vi "add wait(SubVI).vi"(10 "字符串":string) -> (1 "ok or cancel":bool, 2 "连接的字符串":string)   [LabVIEW 2019, in "SubVI.lvlib"]
uses:
  SubVI.lvlib
panel:
  in  "cancel":bool
  in  "ok":bool
  in  "Delay(secs)":dbl
  in  "Chamber":bool
  in  "Position":bool
  in  "Field":bool
  in  "Temperature":bool
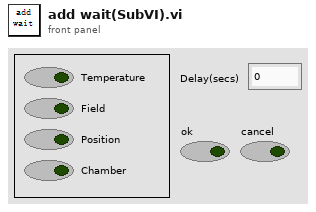
[diagram p1: front panel]
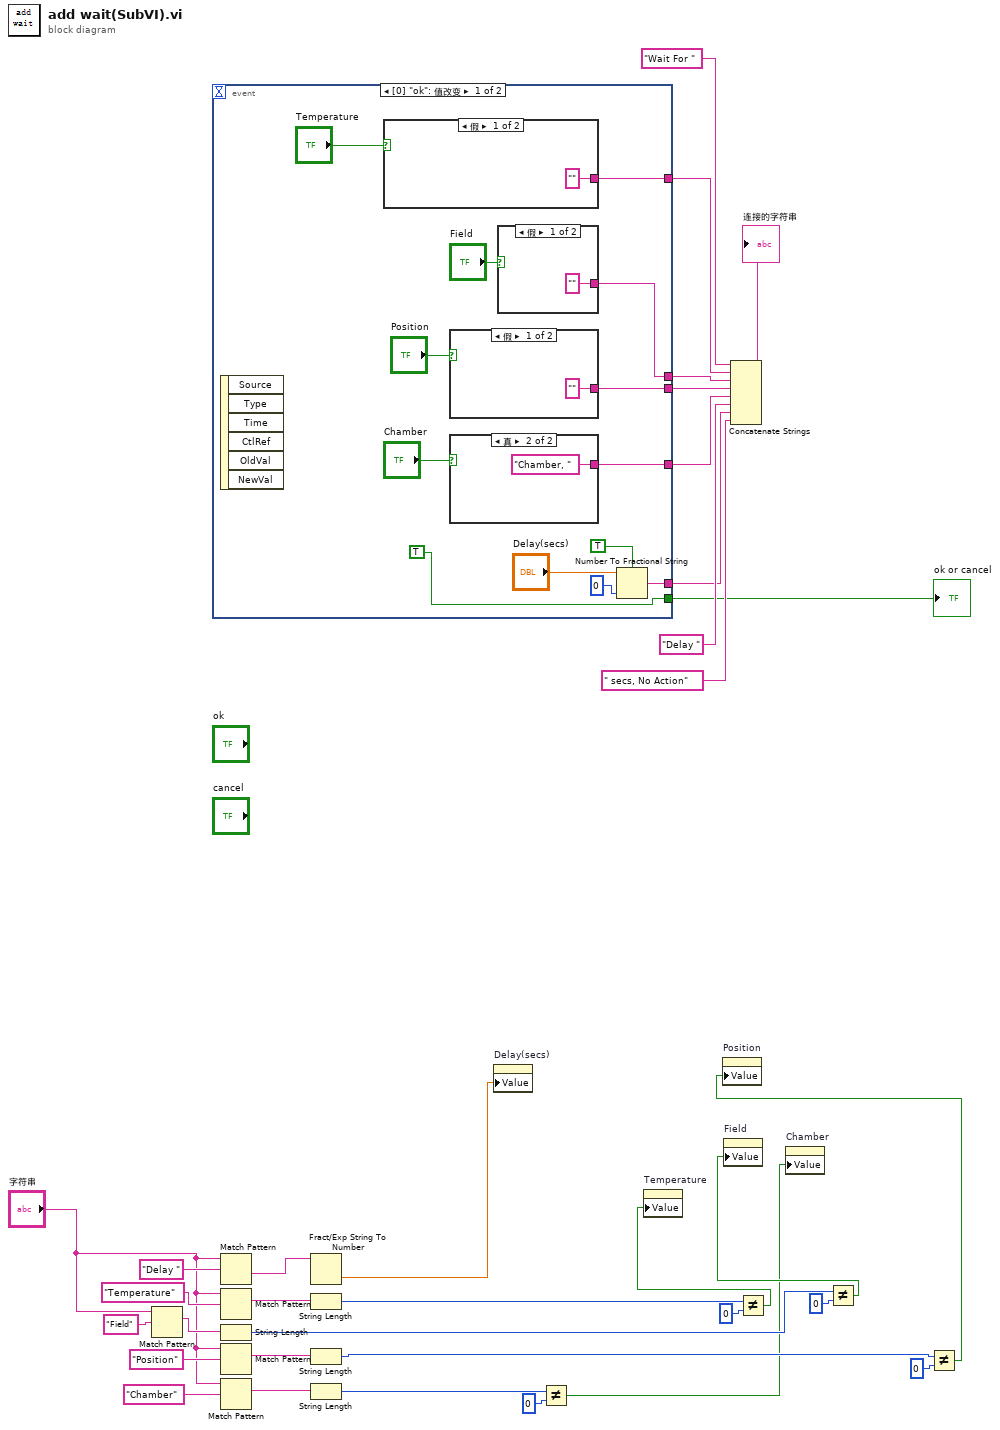
[diagram p0: block diagram]
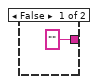
[diagram p2: hidden frame]
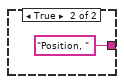
[diagram p3: hidden frame]
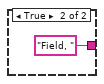
[diagram p4: hidden frame]
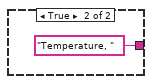
[diagram p5: hidden frame]
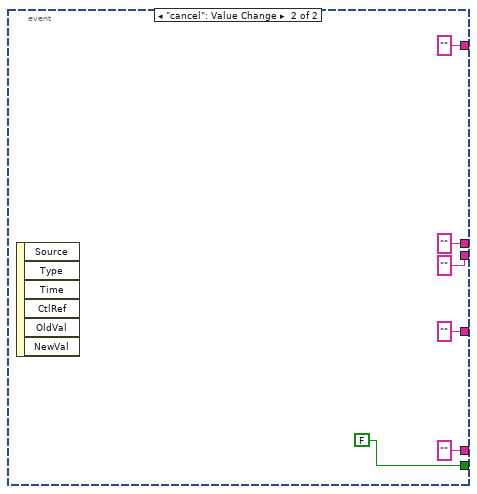
[diagram p6: hidden frame]
diagram:
  n1 = Match Pattern(string="字符串", regular expression="Field" ("正则表达式")) -> (match substring=w21:string)  [unwired: 1 in, 3 out]
  n2 = event shown="[0] \"ok\": 值改变" {
    selector: _ -> [_ _]
    dyn-events: _ -> [_ _]
    timeout: _ -> [_ _]
    tunnel: [w43 ""] -> w33
    tunnel: [w42 ""] -> w32
    tunnel: [w41 ""] -> w31
    tunnel: [w40 ""] -> w30
    tunnel: [w36 ""] -> w28
    tunnel: [TRUE FALSE] -> w26
    event "ok": Value Change {
      n3 = event-data() -> ()  [unwired: 1 in, 6 out]
      n4 = case shown="假" "Temperature" {
        tunnel: ["" "Temperature, "] -> w43
        frame False {
        }
        frame True {
        }
      }
      n5 = case shown="假" "Position" {
        tunnel: ["" "Position, "] -> w41
        frame False {
        }
        frame True {
        }
      }
      n6 = case shown="真" "Chamber" {
        tunnel: ["" "Chamber, "] -> w40
        frame False {
        }
        frame True {
        }
      }
      n7 = case shown="假" "Field" {
        tunnel: ["" "Field, "] -> w42
        frame False {
        }
        frame True {
        }
      }
      n8 = Number To Fractional String(use system decimal point (T)=TRUE ("使用系统小数点(T)"), number="Delay(secs)", precision (6)=i16 0 ("精度(6)")) -> (F-format string=w36:string)  [unwired: 1 in]
    }
    event "cancel": Value Change {
      n9 = event-data() -> ()  [unwired: 1 in, 6 out]
    }
  }
  "ok or cancel" <- w26
  n10 = Match Pattern(string="字符串", regular expression="Delay " ("正则表达式")) -> (after substring=w7:string)  [unwired: 1 in, 3 out]
  n11 = Match Pattern(string="字符串", regular expression="Temperature" ("正则表达式")) -> (match substring=w24:string)  [unwired: 1 in, 3 out]
  n12 = String Length(string=w21) -> (length=w20:i32)
  n13 = Match Pattern(string="字符串", regular expression="Position" ("正则表达式")) -> (match substring=w18:string)  [unwired: 1 in, 3 out]
  n14 = Match Pattern(string="字符串", regular expression="Chamber" ("正则表达式")) -> (match substring=w15:string)  [unwired: 1 in, 3 out]
  n15 = Fract/Exp String To Number(string=w7) -> (number=w5:dbl)  [unwired: 3 in, 1 out]
  n16 = String Length(string=w24) -> (length=w23:i32)
  n17 = String Length(string=w18) -> (length=w17:i32)
  n18 = String Length(string=w15) -> (length=w14:i32)
  n19 = property on="Delay(secs)" class="DigNum (严格)"("Value"=w5) -> ()  [unwired: 2 in, 2 out]
  n20 = Not Equal?(x=w14, y=0) -> (x != y?=w1:bool)
  n21 = Concatenate Strings("Wait For " ("字符串"), w33, w32, w31, w30, "Delay " ("字符串"), w28, " secs, No Action" ("字符串")) -> (→"连接的字符串":string)
  n22 = Not Equal?(x=w23, y=0) -> (x != y?=w4:bool)
  n23 = property on="Temperature" class="Bool (严格)"("Value"=w4) -> ()  [unwired: 2 in, 2 out]
  n24 = property on="Chamber" class="Bool (严格)"("Value"=w1) -> ()  [unwired: 2 in, 2 out]
  n25 = Not Equal?(x=w20, y=0) -> (x != y?=w3:bool)
  n26 = property on="Field" class="Bool (严格)"("Value"=w3) -> ()  [unwired: 2 in, 2 out]
  n27 = Not Equal?(x=w17, y=0) -> (x != y?=w2:bool)
  n28 = property on="Position" class="Bool (严格)"("Value"=w2) -> ()  [unwired: 2 in, 2 out]
